vi "Read Holding Registers.vi"(7 "unit ID":u8, 8 "error in":errorcluster, 9 "number of inputs":u16, 10 "starting address":u16, 11 "Modbus master in":refnum<class "Modbus Master.lvclass">) -> (0 "error out":errorcluster, 2 "register values":u16[](array[numeric]), 3 "Modbus master out":refnum<class "Modbus Master.lvclass">)   [LabVIEW 2013, in "Modbus Library - Advance.lvlib" / "Modbus Master.lvclass"]
doc: "Reads <B>number of inputs</B> holding registers starting at <B>starting address</B> from the device."
uses:
  Modbus Master.lvclass
  Modbus Master.lvclass/Modbus Master.ctl
  Modbus API.lvclass/Modbus API.ctl
  Transmission Data Unit/Transmission Data Unit.lvclass/Transmission Data Unit.ctl
  Transmission Data Unit/Transmission Data Unit.lvclass
  Modbus API.lvclass
  Master Function Definition/Master Function Definition.lvclass
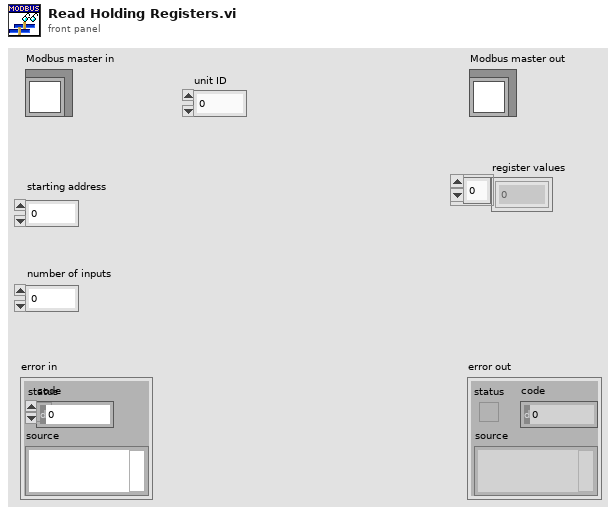
[diagram p1: front panel]
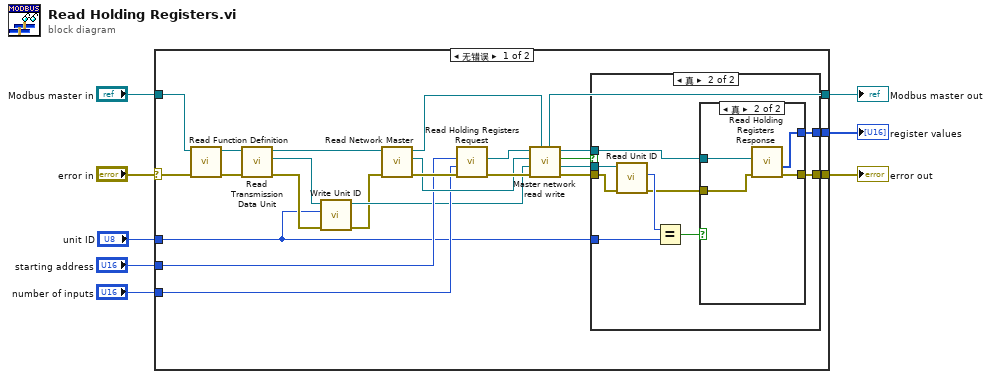
[diagram p0: block diagram]
diagram:
  n1 = case shown="无错误" "error in" {
    selector: "error in" -> [w29 w48]
    tunnel: "number of inputs" -> [w19 _]
    tunnel: "starting address" -> [w20 _]
    tunnel: "Modbus master in" -> [w28 w49]
    tunnel: [w23 w49] -> w4
    tunnel: [w24 w48] -> w3
    tunnel: [w18 _] -> w2
    tunnel: "unit ID" -> [w9 _]
    frame No Error {
      n2 = call "Read Function Definition.vi"("error in"=w29, "Modbus master in"=w28) -> ("error out"=w31:errorcluster, "Modbus master out"=w32:refnum<class "Modbus Master.lvclass">)  [unwired: 7 in, 1 out]
      n3 = call "Read Transmission Data Unit.vi"("error in"=w31, "Modbus instance in"=w32) -> ("error out"=w12:errorcluster, "transmission data unit"=w14:refnum<class "Transmission Data Unit.lvclass">, "Modbus instance out"=w30:refnum<class "Modbus Master.lvclass">)  [unwired: 7 in]
      n4 = call "Write Unit ID.vi"("error in"=w12, "unit ID"=w9, "transmission data unit in"=w14) -> ("error out"=w11:errorcluster, "transmission data unit out"=w13:refnum<class "Transmission Data Unit.lvclass">)  [unwired: 7 in]
      n5 = call "Read Network Master.vi"("error in"=w11, "Modbus master in"=w30) -> ("error out"=w25:errorcluster, "network master"=w21:refnum<class "Network Master.lvclass">, "Modbus master out"=w22:refnum<class "Modbus Master.lvclass">)  [unwired: 7 in]
      n6 = call "Read Holding Registers Request.vi"("error in"=w25, "Number of Registers"=w19, "Starting Address"=w20) -> ("error out"=w26:errorcluster, "modbus data unit out"=w16:refnum<class "Modbus Data Unit.lvclass">)  [unwired: 7 in]
      n7 = call "Master network read write.vi"("Modbus master in"=w22, "error in"=w26, "transmission data unit in"=w13, "network master in"=w21, "Modbus data unit in"=w16) -> ("error out"=w27:errorcluster, "transmission data unit out"=w10:refnum<class "Transmission Data Unit.lvclass">, "PDU Valid?"=w15:bool, "Modbus data unit out"=w17:refnum<class "Modbus Data Unit.lvclass">, "Modbus master out"=w23:refnum<class "Modbus Master.lvclass">)  [unwired: 2 in]
      n8 = case shown="真" w15 {
        tunnel: w27 -> [w33 w38]
        tunnel: [w33 w42] -> w24
        tunnel: [_ w41] -> w18
        tunnel: w17 -> [_ w40]
        tunnel: w10 -> [_ w39]
        tunnel: w9 -> [_ w36]
        frame False {
        }
        frame True {
          n9 = call "Read Unit ID.vi"("error in"=w38, "transmission data unit in"=w39) -> ("error out"=w34:errorcluster, "unit ID"=w37:u8)  [unwired: 7 in, 1 out]
          n10 = Equal?(x=w37, y=w36) -> (x = y?=w35:bool)
          n11 = case shown="真" w35 {
            tunnel: [w43 w47] -> w42
            tunnel: [_ w46] -> w41
            tunnel: w40 -> [_ w45]
            tunnel: w34 -> [w43 w44]
            frame False {
            }
            frame True {
              n12 = call "Read Holding Registers Response.vi"("error in"=w44, "modbus data unit in"=w45) -> ("error out"=w47:errorcluster, "Register Values"=w46:u16[])  [unwired: 7 in, 1 out]
            }
          }
        }
      }
    }
    frame Error {
    }
  }
  "Modbus master out" <- w4
  "error out" <- w3
  "register values" <- w2
